vi "SetupQueue.vi"(0 "Cmd":string, 1 "Value":string, 3 "Queue in":refnum<queue>) -> (2 "Cluster":cluster{"Cmd":string, "Value":string}, 5 "Queue out":refnum<queue>)   [LabVIEW 2015]
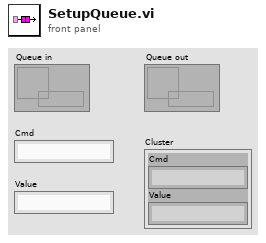
[diagram p1: front panel]
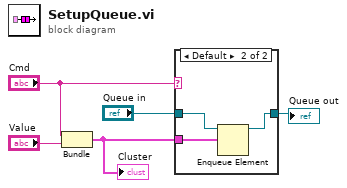
[diagram p0: block diagram]
diagram:
  n1 = Bundle("Cmd"="Cmd", "Value"="Value") -> (w5:cluster{"Cmd":string, "Value":string})  [unwired: 1 in]
  "Cluster" <- w5
  n2 = case shown="Default" "Cmd" {
    tunnel: w5 -> [_ w9]
    tunnel: [w6 w8] -> w3
    tunnel: "Queue in" -> [w6 w7]
    frame "" {
    }
    frame Default {
      n3 = Enqueue Element(queue=w7, element=w9) -> (queue out=w8:refnum<queue>)  [unwired: 2 in, 2 out]
    }
  }
  "Queue out" <- w3
